vi "Main On Compile Action VI_Prepare Async_RTs Start Stop Channels.vi"(8 "error in (no error)":errorcluster, 10 "channels":T3[](array[typedef]) {"RTs"."Mode Codes"."Words Item Refs" format="%.0x"; "RTs"."Mode Codes"."Timestamp Channel Data Reference" format="%.0x"; "RTs"."subAddresses"."Words Item Refs" format="%.0x"; "RTs"."subAddresses"."Timestamp Channel Data Reference" format="%.0x"; "RTs"."Status Channel Data Reference" format="%.0x"; "RTs"."Command Channels Refs" format="%.0x"; "BC"."Acyclic Frames Trigger Channels Refs" format="%.0x"; "BC"."Command Channels Refs" format="%.0x"; "BC"."messages"."Timestamp Channel Data Reference" format="%.0x"; "BC"."messages"."Status Channel Data Refs" format="%.0x"; "BC"."messages"."Words Item Refs" format="%.0x"; "BC"."messages"."Words Block Data Refs"."Data Reference" format="%.0x"}, 11 "Item Ref In":T1 format="%.0x") -> (0 "error out":errorcluster, 1 "Group":T2 {"VS Refs" format="%.0x"}, 2 "channels":T3[](array[typedef]) {"RTs"."Mode Codes"."Words Item Refs" format="%.0x"; "RTs"."Mode Codes"."Timestamp Channel Data Reference" format="%.0x"; "RTs"."subAddresses"."Words Item Refs" format="%.0x"; "RTs"."subAddresses"."Timestamp Channel Data Reference" format="%.0x"; "RTs"."Status Channel Data Reference" format="%.0x"; "RTs"."Command Channels Refs" format="%.0x"; "BC"."Acyclic Frames Trigger Channels Refs" format="%.0x"; "BC"."Command Channels Refs" format="%.0x"; "BC"."messages"."Timestamp Channel Data Reference" format="%.0x"; "BC"."messages"."Status Channel Data Refs" format="%.0x"; "BC"."messages"."Words Item Refs" format="%.0x"; "BC"."messages"."Words Block Data Refs"."Data Reference" format="%.0x"}, 3 "Item Ref Out":T1 format="%.0x")   [LabVIEW 2020, in "Ballard 1553 System Explorer.lvlib"]
uses:
  Ballard 1553 System Explorer.lvlib
  <vilib>/NI VeriStand/Custom Device API/Custom Device Item Ref.ctl
  Shared/Controls and Global/RT Channel.ctl
  Shared/Controls and Global/RT BC.ctl
  Shared/Controls and Global/RT Message.ctl
  Shared/Controls and Global/RT messageType.ctl
  Shared/Controls and Global/RT CWD1.ctl
  Shared/Controls and Global/RT CWD2.ctl
  <vilib>/NI VeriStand/Custom Device API/Data Reference.ctl
  <vilib>/NI VeriStand/Custom Device API/Block Data Reference.ctl
  Shared/Controls and Global/RT Remote Terminal.ctl
  Shared/Controls and Global/RT Remote Terminal_rtMode.ctl
  Shared/Controls and Global/RT Remote Terminal_RT subAddress.ctl
  Shared/Controls and Global/RT Remote Terminal_RT direction.ctl
  Shared/Controls and Global/RT Remote Terminal_RT Mode Code.ctl
  <vilib>/NI VeriStand/Custom Device API/Custom Device API.lvlib
  Shared/Ballard 1553 Shared.lvlib
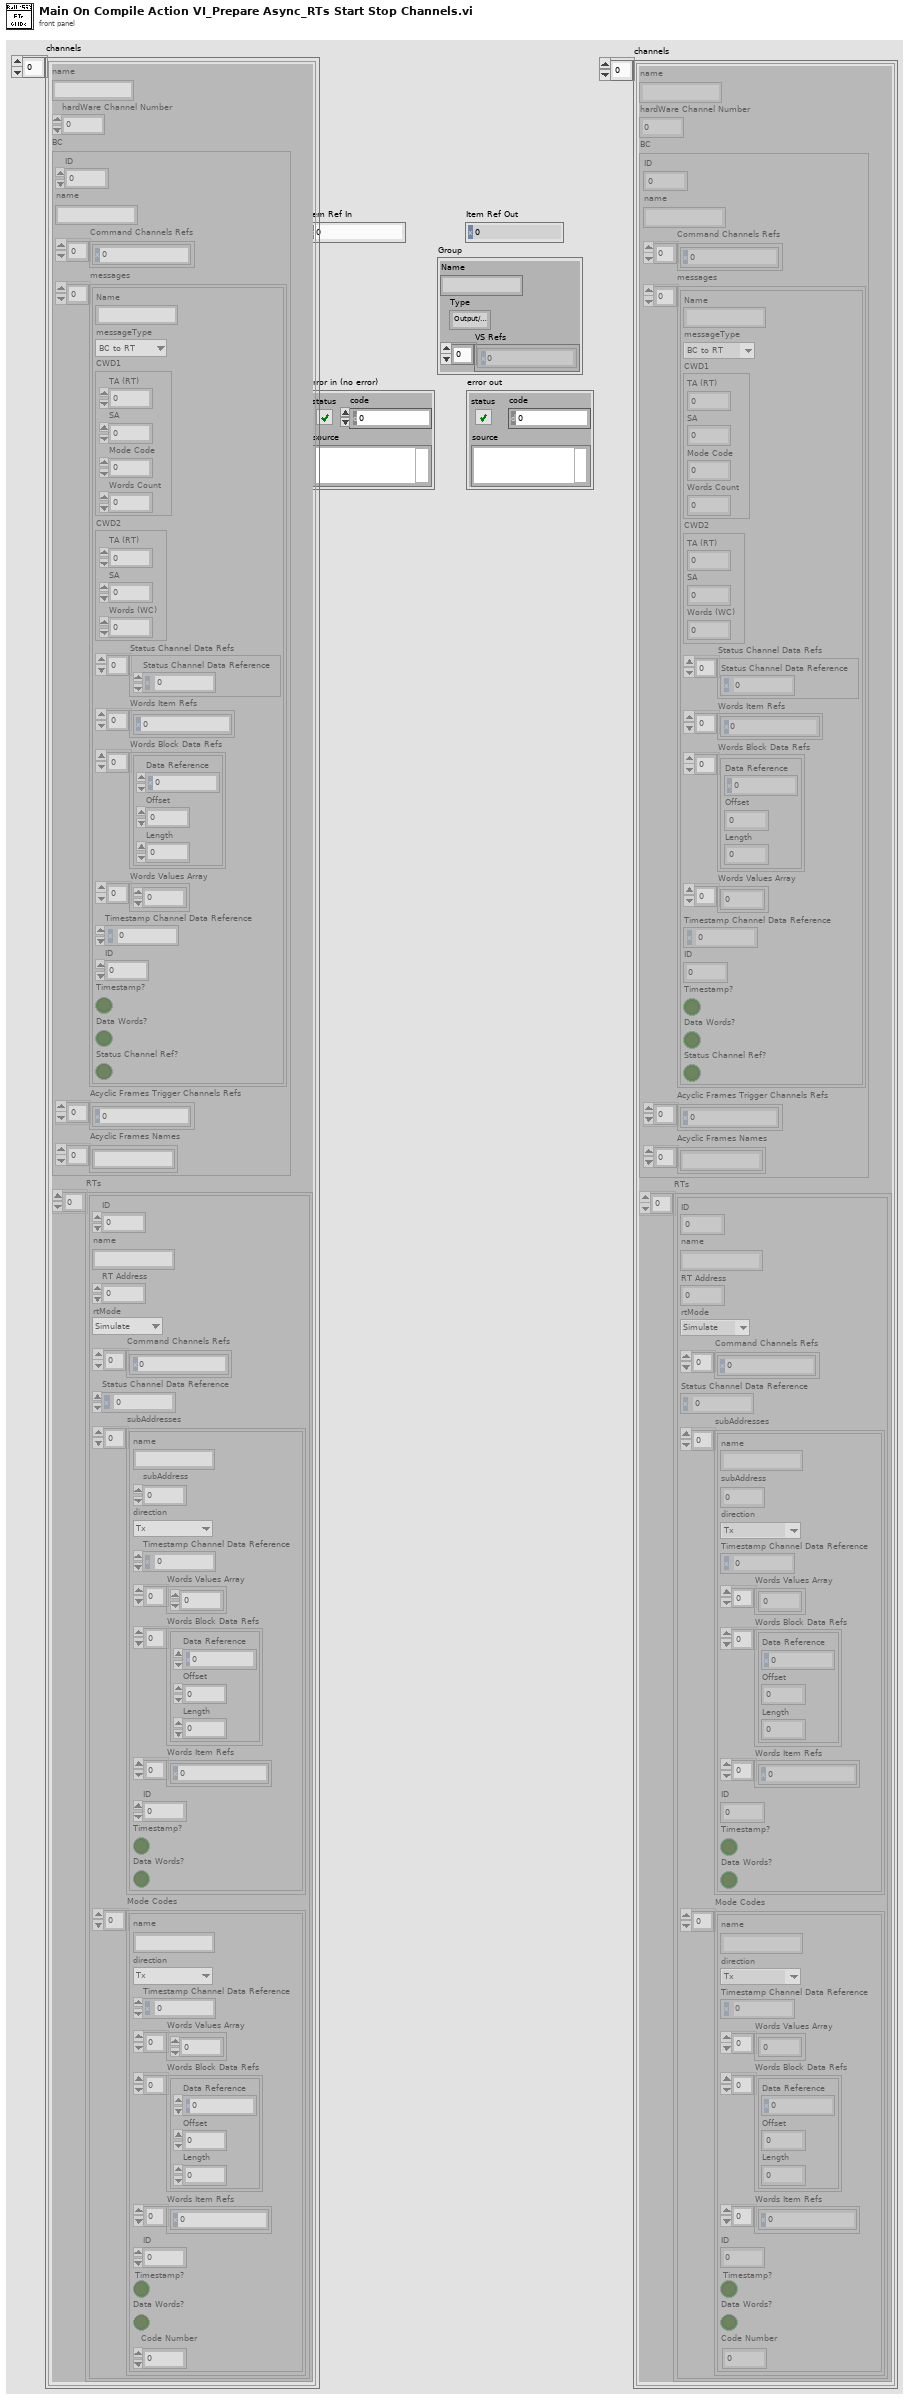
[diagram p1: front panel]
types:
  T1 = typedef "Custom Device API.lvlib/Custom Device Item Ref.ctl" = u64
  T2 = cluster{"Name":string, "Type":enum16{"Output/Write", "Input/Read", "Input/ReadWrite"}, "VS Refs":T1[]}
  T3 = typedef "Ballard 1553 Shared.lvlib/RT Channel.ctl" = cluster{"name":string, "hardWare Channel Number":u16, "BC":T4, "RTs":T11[]}
  T4 = typedef "Ballard 1553 Shared.lvlib/RT BC.ctl" = cluster{"ID":i32, "name":string, "Command Channels Refs":T1[], "messages":T5[], "Acyclic Frames Trigger Channels Refs":T1[], "Acyclic Frames Names":string[]}
  T5 = typedef "Ballard 1553 Shared.lvlib/RT Message.ctl" = cluster{"Name":string, "messageType":T6, "CWD1":T7, "CWD2":T8, "Status Channel Data Refs":T9[], "Words Item Refs":T1[], "Words Block Data Refs":T10[], "Words Values Array":u16[], "Timestamp Channel Data Reference":T9, "ID":i32, "Timestamp?":bool, "Data Words?":bool, "Status Channel Ref?":bool}
  T6 = typedef "Ballard 1553 Shared.lvlib/RT messageType.ctl" = enum16{"BC to RT", "RT to BC", "RT to RT", "MC (Rx)", "MC (Tx)"}
  T7 = typedef "Ballard 1553 Shared.lvlib/RT CWD1.ctl" = cluster{"TA (RT)":i8, "SA":i8, "Mode Code":i8, "Words Count":i8}
  T8 = typedef "Ballard 1553 Shared.lvlib/RT CWD2.ctl" = cluster{"TA (RT)":i8, "SA":i8, "Words (WC)":i8}
  T9 = typedef "Custom Device API.lvlib/Data Reference.ctl" = i32
  T10 = typedef "Custom Device API.lvlib/Block Data Reference.ctl" = cluster{"Data Reference":T9, "Offset":u64, "Length":u64}
  T11 = typedef "Ballard 1553 Shared.lvlib/RT Remote Terminal.ctl" = cluster{"ID":i32, "name":string, "RT Address":i32, "rtMode":T12, "Command Channels Refs":T1[], "Status Channel Data Reference":T9, "subAddresses":T13[], "Mode Codes":T15[]}
  T12 = typedef "Ballard 1553 Shared.lvlib/RT Remote Terminal_rtMode.ctl" = enum16{"Simulate", "Monitor", "Disable"}
  T13 = typedef "Ballard 1553 Shared.lvlib/RT Remote Terminal_RT subAddress.ctl" = cluster{"name":string, "subAddress":i8, "direction":T14, "Timestamp Channel Data Reference":T9, "Words Values Array":u16[], "Words Block Data Refs":T10[], "Words Item Refs":T1[], "ID":i32, "Timestamp?":bool, "Data Words?":bool}
  T14 = typedef "Ballard 1553 Shared.lvlib/RT Remote Terminal_RT direction.ctl" = enum16{"Tx", "Rx"}
  T15 = typedef "Ballard 1553 Shared.lvlib/RT Remote Terminal_RT Mode Code.ctl" = cluster{"name":string, "direction":T14, "Timestamp Channel Data Reference":T9, "Words Values Array":u16[], "Words Block Data Refs":T10[], "Words Item Refs":T1[], "ID":i32, "Timestamp?":bool, "Data Words?":bool, "Code Number":i32}
  T16 = enum16{"Output/Write", "Input/Read", "Input/ReadWrite"}
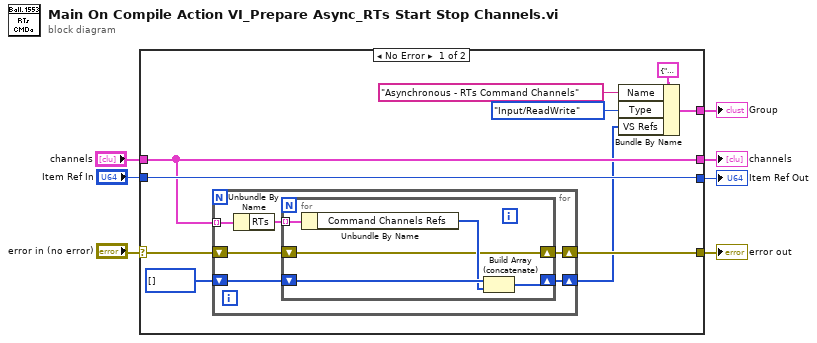
[diagram p0: block diagram]
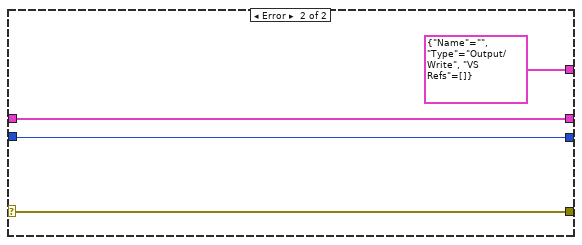
[diagram p2: hidden frame]
diagram:
  n1 = case shown="No Error" "error in (no error)" {
    selector: "error in (no error)" -> [w16 w32]
    tunnel: "Item Ref In" -> [w17 w31]
    tunnel: [w14 w32] -> w5
    tunnel: "channels" -> [w15 w30]
    tunnel: [w15 w30] -> w3
    tunnel: [w17 w31] -> w2
    tunnel: [w10 T2 {"Name"="", "Type"=enum."Output/Write", "VS Refs"=[]} ("Group")] -> w1
    frame No Error {
      n2 = for {
        tunnel: w15 -> [w23] mode=indexing
        shift-right: [w18] -> w14
        shift-left: w16 -> [w20]
        shift-right: [w21] -> w11
        shift-left: T1[] [] -> [w22]
        n3 = Unbundle By Name(w23) -> ("RTs"=w19:T11[])
        n4 = for {
          shift-right: [w27] -> w21
          shift-left: w22 -> [w28]
          shift-right: [w24] -> w18
          shift-left: w20 -> [w24]
          tunnel: w19 -> [w26] mode=indexing
          n5 = Unbundle By Name(w26) -> ("Command Channels Refs"=w25:T1[])
          n6 = Build Array (concatenate)(w28, w25) -> (w27:T1[])
        }
      }
      n7 = Bundle By Name(cluster=T2 {"Name"="", "Type"=enum."Output/Write", "VS Refs"=[]} ("Group"), "Name"="Asynchronous - RTs Command Channels", "Type"=T16."Input/ReadWrite", "VS Refs"=w11) -> (w10:T2)
    }
    frame Error {
    }
  }
  "error out" <- w5
  "Item Ref Out" <- w2
  "channels" <- w3
  "Group" <- w1
